vi "RemovedDuplicateCommands.vi"(5 "Timeout (ms)":i32=-1, 7 "Search for Command":string, 8 "error in (no error)":errorcluster, 9 "Data - IN":variant, 10 "Arguments - IN":string[](array[string]), 11 "Queue In":T1) -> (0 "error out":errorcluster, 1 "Data - OUT":variant, 2 "Arguments - OUT":string[](array[string]), 3 "queue (dup)":T1)   [LabVIEW 2010]
doc: "This VI serves to dequeue a command from the string queue provided to the input. The queue sorts the command from the command line arguements, which can be included after the command. The arguements are separated by a colon (:) and will be output as a string array. The VI will also handle any error that exists in the error cluster by setting the command = Error with the error code and error string message as arguments.\n\nInputs:\nqueue - input queue (string)\nTimeout (ms) - timeout (in milliseconds) for the dequeue function to wait (default -1 = no timeout)\nerror in - error input cluster\n\nOutputs:\ncommand - main state in the queue; this is used as the current state to be used by the case structure\narguments - command line arguments that were included with the command; separated by colon (:)\nqueue - duplicate reference for the queue\nerror out - error output cluster"
uses:
  <userlib>/Common/Queue with Cluster/TYP_Queue with Cluster Reference.ctl
panel:
  out "# elements in queue":i32
  out "Duplicate Count":i32
  # "Inputs"
  # "Local"
  # "Outputs"
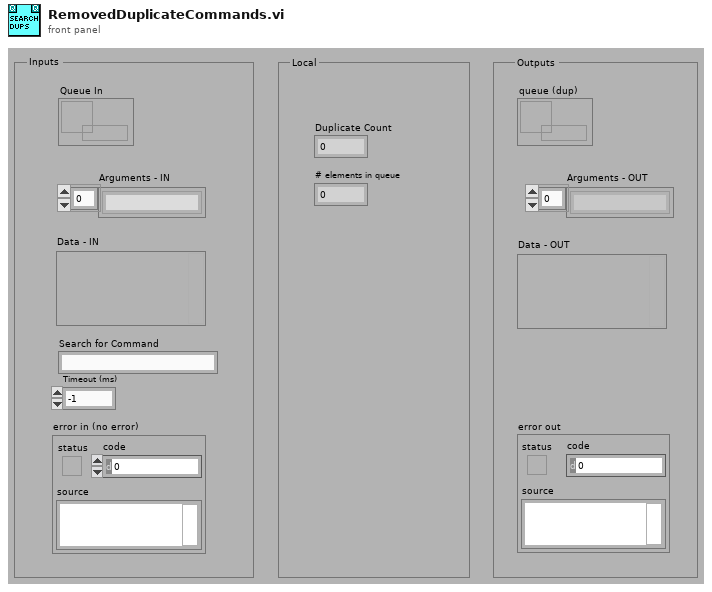
[diagram p1: front panel]
types:
  T1 = typedef "TYP_Queue with Cluster Reference.ctl" = refnum<queue>
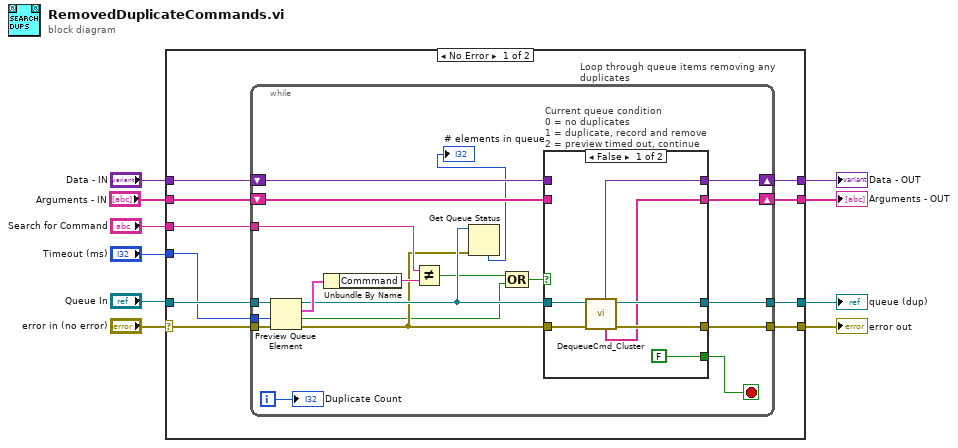
[diagram p0: block diagram]
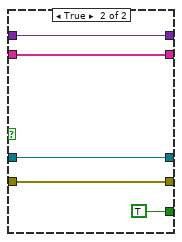
[diagram p2: hidden frame]
diagram:
  n1 = case shown="No Error" "error in (no error)" {
    selector: "error in (no error)" -> [w19 w55]
    tunnel: [w15 w55] -> w10
    tunnel: "Queue In" -> [w20 w56]
    tunnel: [w16 w56] -> w7
    tunnel: "Timeout (ms)" -> [w18 _]
    tunnel: "Search for Command" -> [w17 _]
    tunnel: "Data - IN" -> [w14 w54]
    tunnel: "Arguments - IN" -> [w13 w53]
    tunnel: [w12 w54] -> w3
    tunnel: [w11 w53] -> w1
    frame No Error {
      n2 = while "Loop through queue items removing any duplicates" {
        tunnel: w20 -> [w40]
        tunnel: w19 -> [w39]
        tunnel: w18 -> [w38]
        tunnel: w17 -> [w35]
        tunnel: [w34] -> w16
        tunnel: [w33] -> w15
        shift-right: [w32] -> w12
        shift-left: w14 -> [w30]
        shift-right: [w31] -> w11
        shift-left: w13 -> [w29]
        i -> [w27]
        stop <- w28 stop-if-true
        n3 = Preview Queue Element(queue=w40, timeout in ms (-1)=w38, error in (no error)=w39) -> (queue out=w26:T1, element=w37:cluster{"Commmand":string, "Data":variant}, timed out?=w22:bool, error out=w25:errorcluster)
        n4 = Unbundle By Name(w37) -> ("Commmand"=w36:string)
        n5 = Not Equal?(x=w35, y=w36) -> (x != y?=w21:bool)
        n6 = Get Queue Status(queue=w26, error in (no error)=w25) -> (# elements in queue=→"# elements in queue":i32)  [unwired: 1 in, 7 out]
        n7 = Compound Arithmetic op=OR(w21, w22) -> (w23:bool)
        n8 = case "Current queue condition\n0 = no duplicates\n1 = duplicate, record and remove\n2 = preview timed out, continue" shown="False" w23 {
          tunnel: w26 -> [w46 w50]
          tunnel: w25 -> [w45 w49]
          tunnel: [w44 w50] -> w34
          tunnel: [w43 w49] -> w33
          tunnel: [FALSE TRUE] -> w28
          tunnel: [w42 w52] -> w32
          tunnel: [w41 w51] -> w31
          tunnel: w30 -> [_ w52]
          tunnel: w29 -> [_ w51]
          frame False {
            n9 = call <userlib>:"DequeueCmd_Cluster.vi"("error in (no error)"=w45, "Queue In"=w46) -> ("error out"=w43:errorcluster, "queue (dup)"=w44:T1, "arguments"=w41:string[], "Data"=w42:variant)  [unwired: 4 in, 2 out]
          }
          frame True {
          }
        }
        "Duplicate Count" <- w27
      }
    }
    frame Error {
    }
  }
  "error out" <- w10
  "queue (dup)" <- w7
  "Data - OUT" <- w3
  "Arguments - OUT" <- w1
